vi "Initialize.vi"(0 "Simulated Power Meter in":refnum<class "Simulated Power Meter.lvclass">, 11 "error in (no error)":errorcluster) -> (4 "Simulated Power Meter out":refnum<class "Simulated Power Meter.lvclass">, 15 "error out":errorcluster)   [LabVIEW 2023, in "RFFixtureCharact.Instruments.lvlib" / "Simulated Power Meter.lvclass"]
uses:
  Simulated Power Meter.lvclass
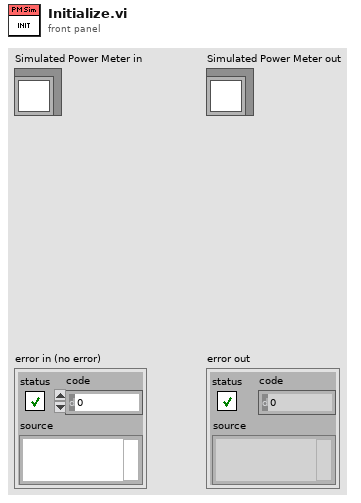
[diagram p1: front panel]
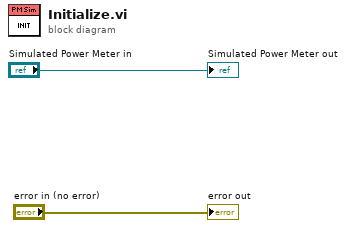
[diagram p0: block diagram]
diagram:
  "error out" <- "error in (no error)"
  "Simulated Power Meter out" <- "Simulated Power Meter in"
